vi "WPI_SimpleGyroGlobal.vi"() -> ()   [LabVIEW 2014, in "SimpleGyro.lvlib"]
uses:
  SimpleGyro.lvlib
panel:
  in  "Gyro Reset":bool
  in  "Gyro Angle":dbl
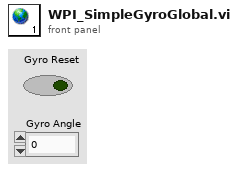
[diagram p1: front panel]
diagram:
